vi "Pick_diagnostics.vi"(2 "error in (no error)":errorcluster, 3 "Data In":T1) -> (0 "error out":errorcluster, 1 "Data Out":T1)   [LabVIEW 2015, in "Steps.lvlib"]
uses:
  Steps.lvlib
  Data.ctl
  Diagnostics.ctl
  Systems.ctl
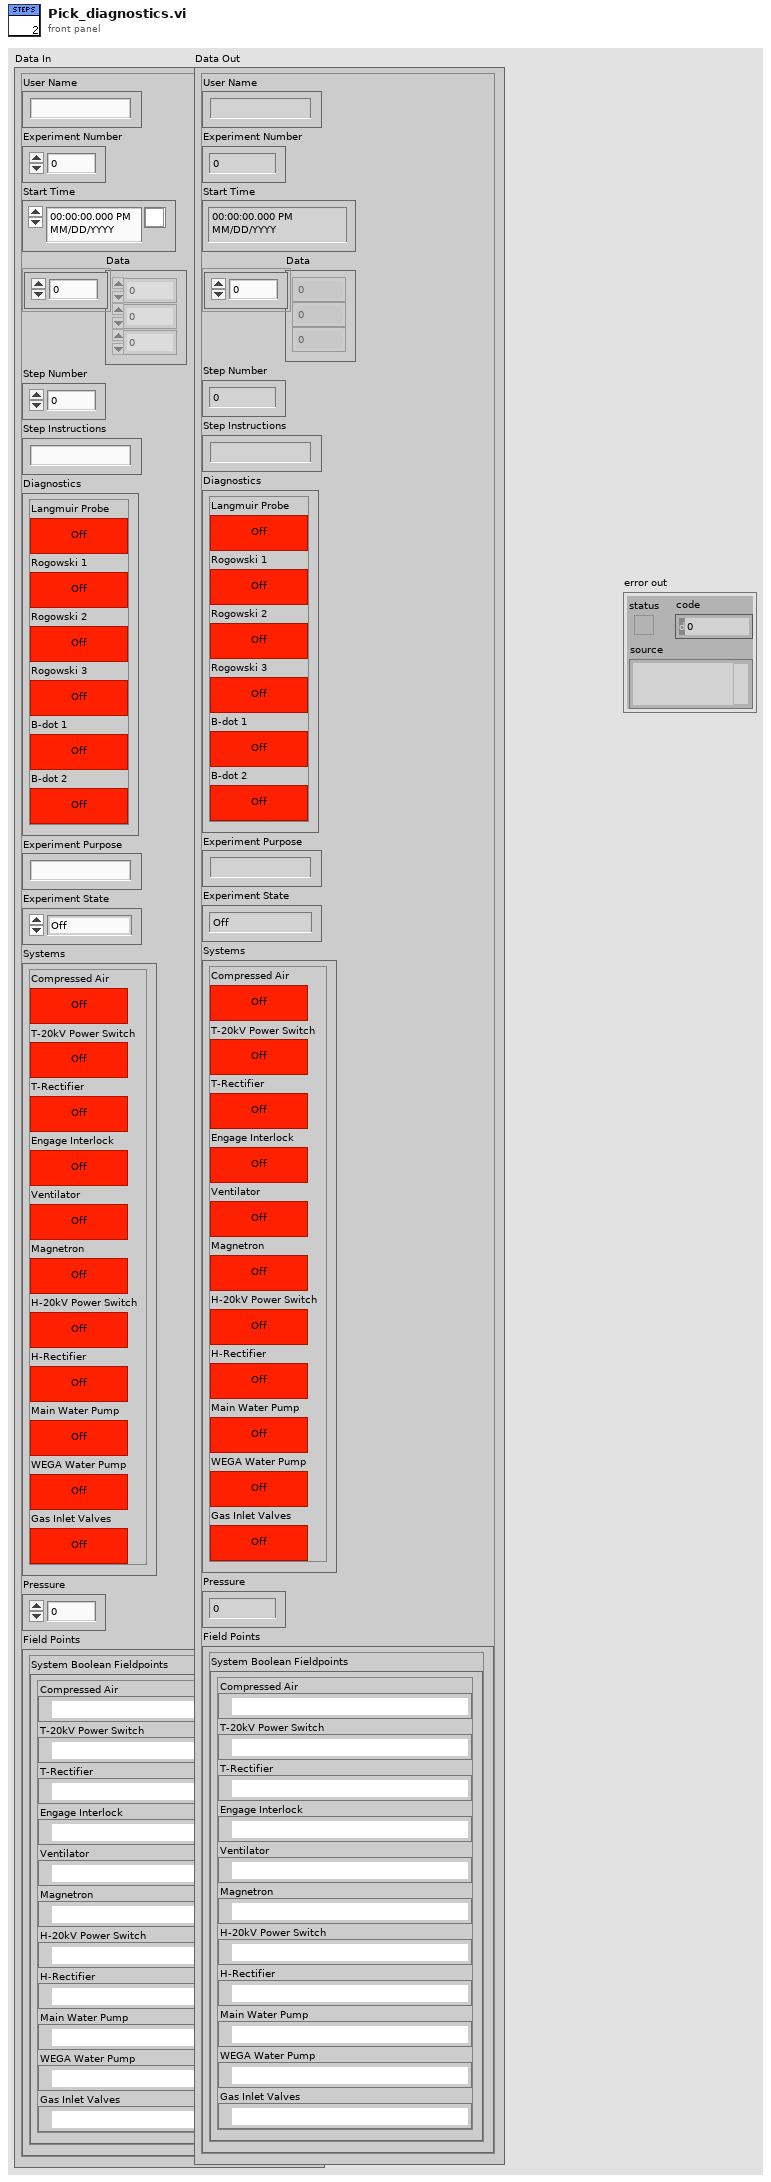
[diagram p1: front panel]
types:
  T1 = typedef "Data.ctl" = cluster{"User Name":string, "Experiment Number":i32, "Start Time":timestamp, "Data":dbl[], "Step Number":i32, "Step Instructions":string, "Diagnostics":T2, "Experiment Purpose":string, "Experiment State":enum16{"Off", "Setting Up", "Ready", "In Progress", "Shutting Down"}, "Systems":T3, "Pressure":dbl, "Field Points":cluster{"System Boolean Fieldpoints":cluster{"Compressed Air":refnum<k21>, "T-20kV Power Switch":refnum<k21>, "T-Rectifier":refnum<k21>, "Engage Interlock":refnum<k21>, "Ventilator":refnum<k21>, "Magnetron":refnum<k21>, "H-20kV Power Switch":refnum<k21>, "H-Rectifier":refnum<k21>, "Main Water Pump":refnum<k21>, "WEGA Water Pump":refnum<k21>, "Gas Inlet Valves":refnum<k21>}}}
  T2 = typedef "Diagnostics.ctl" = cluster{"Langmuir Probe":bool, "Rogowski 1":bool, "Rogowski 2":bool, "Rogowski 3":bool, "B-dot 1":bool, "B-dot 2":bool}
  T3 = typedef "Systems.ctl" = cluster{"Compressed Air":bool, "T-20kV Power Switch":bool, "T-Rectifier":bool, "Engage Interlock":bool, "Ventilator":bool, "Magnetron":bool, "H-20kV Power Switch":bool, "H-Rectifier":bool, "Main Water Pump":bool, "WEGA Water Pump":bool, "Gas Inlet Valves":bool}
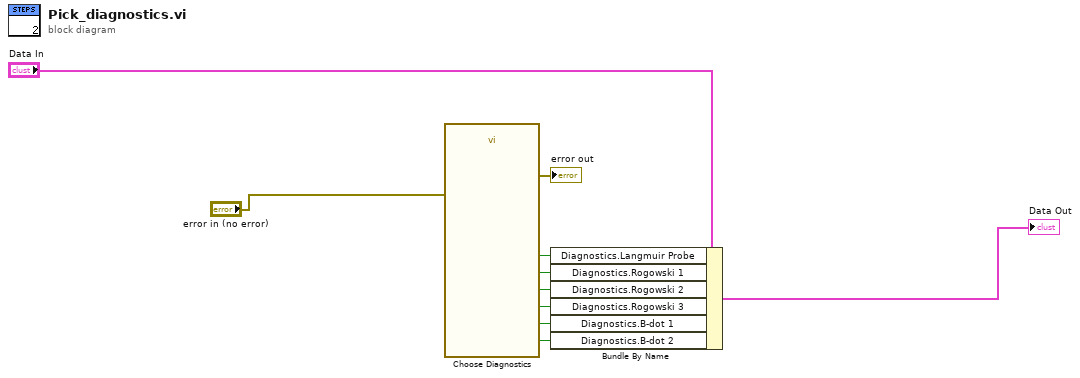
[diagram p0: block diagram]
diagram:
  n1 = call "Choose Diagnostics"("error in (no error)"="error in (no error)") -> ("B-dot 2"=w4:bool, "B-dot 1"=w5:bool, "Rogowski 3"=w3:bool, "Rogowski 2"=w6:bool, "Rogowski 1"=w7:bool, "Langmuir Probe"=w8:bool, "error out"=→"error out":errorcluster)  [unwired: 11 in, 1 out]
  n2 = Bundle By Name(cluster="Data In", "Diagnostics.Langmuir Probe"=w8, "Diagnostics.Rogowski 1"=w7, "Diagnostics.Rogowski 2"=w6, "Diagnostics.Rogowski 3"=w3, "Diagnostics.B-dot 1"=w5, "Diagnostics.B-dot 2"=w4) -> (→"Data Out":T1)
